vi "ReadFontStyle.vi"(7 "Dictionary":string[][](array[string]), 8 "error in (no error)":errorcluster, 10 "Target Language":string) -> (0 "error out":errorcluster, 2 "Font Info":T1)   [LabVIEW 2017, in "JKI Simple Localization.lvlib"]
uses:
  API/JKI Simple Localization.lvlib
  Definitions/Font Info.ctl
  <userlib>/_OpenG.lib/error/error.llb/Filter Error Codes (Array)__ogtk.vi
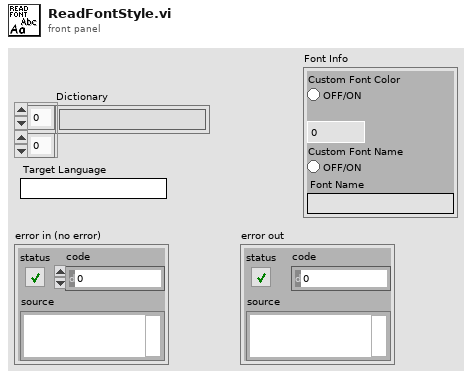
[diagram p1: front panel]
types:
  T1 = typedef "JKI Simple Localization.lvlib/Font Info.ctl" = cluster{"Custom Font Color":bool, "Font Color":u32, "Custom Font Name":bool, "Font Name":string}
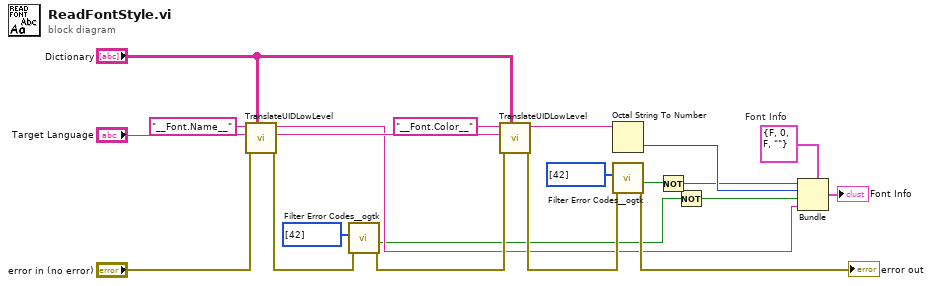
[diagram p0: block diagram]
diagram:
  w6 = T1 {"Custom Font Color"=FALSE, "Font Color"=0, "Custom Font Name"=FALSE, "Font Name"=""}  # Font Info
  n1 = call "TranslateUIDLowLevel.vi"("Dictionary"="Dictionary", "error in (no error)"="error in (no error)", "Target Language"="Target Language", "UID"="__Font.Name__") -> ("error out"=w14:errorcluster, "Translated Word"=w8:string)  [unwired: 6 in]
  n2 = call-poly <userlib>:"Filter Error Codes__ogtk.vi"("Error In"=w14, "Error Codes to Filter"=i32[] [42]) -> ("Error Out"=w16:errorcluster, "Error Filtered?"=w2:bool)  [unwired: 7 in, 1 out]
  n3 = call "TranslateUIDLowLevel.vi"("Dictionary"="Dictionary", "error in (no error)"=w16, "Target Language"="Target Language", "UID"="__Font.Color__") -> ("error out"=w19:errorcluster, "Translated Word"=w10:string)  [unwired: 6 in]
  n4 = Octal String To Number(4:w10) -> (0:w7:u32)  [unwired: 2 in, 1 out]
  n5 = call-poly <userlib>:"Filter Error Codes__ogtk.vi"("Error In"=w19, "Error Codes to Filter"=i32[] [42]) -> ("Error Out"=→"error out":errorcluster, "Error Filtered?"=w4:bool)  [unwired: 7 in, 1 out]
  n6 = Not(x=w4) -> (.not. x?=w3:bool)
  n7 = Not(x=w2) -> (.not. x?=w1:bool)
  n8 = Bundle(cluster=w6, "Custom Font Color"=w3, "Font Color"=w7, "Custom Font Name"=w1, "Font Name"=w8) -> (→"Font Info":T1)
